vi "[FPGA] DeltaSig and SARs Main.vi"() -> ()   [LabVIEW 2025]
doc: "This VI provides a template for customizing a waveform acquisition using delta-sigma based NI C Series analog input smodules."
uses:
  <vilib>/eio/EIONode/EIONode.xnode
  <vilib>/eio/EIOPropertyNode/EIOPropertyNode.xnode
  <vilib>/rvi/DataTransferAndStorage/Container/XNode/niFpgaContainer.xnode
  <vilib>/rvi/eio/common/nirviEmuTemplateMethod_errors.vi
  <vilib>/LabVIEW Targets/FPGA/cRIO/shared/nicrio_DsaDataRateApi/_nicrio_9234GetDataRate131.vi
  <vilib>/rvi/interface/RandomDataEmulation/nirviRandomDataFpgaReadWriteTemplate.vi
  <vilib>/LabVIEW Targets/FPGA/cRIO/shared/nicrio_ModuleControls/nicrio_cRIO-9234_DataRatesRing2.ctl
  <vilib>/rvi/eio/common/nirviEmuTemplatePropertyGet_errors.vi
  <vilib>/rvi/eio/common/nirviEmuTemplatePropertyGet_noerrors.vi
  <vilib>/rvi/eio/common/nirviEmuTemplatePropertySet_errors.vi
  <vilib>/rvi/eio/common/nirviEmuTemplatePropertySet_noerrors.vi
panel:
  out "oclk freq":u32
  out "oclk div":u32
  out "oclk mult":u32
  in  "data rate (S/s)":u32
  in  "Chan Scale Array":sgl[](array[numeric])=[0.0, 0.0, 0.0, 0.0, 0.0, 0.0, 0.0, 0.0, 0.0, 0.0, 0.0, 0.0, 0.0, 0.0, 0.0, 0.0, 0.0, 0.0, 0.0, 0.0, 0.0, 0.0, 0.0, 0.0, 0.0, 0.0, 0.0, 0.0, 0.0, 0.0, 0.0, 0.0, 0.0, 0.0, 0.0, 0.0, 0.0, 0.0, 0.0, 0.0]
  out "Chan Count":bool
  out "Acq Loop Ticks":u32
  out "FPGA Error":errorcluster
  out "Module Underflow":bool
  out "Finished":bool
  in  "Number of Channels":i32=4
  in  "Samps per Chan [Finite]":i32=5120
  out "First Read":bool
  in  "Acquisition Type":enum16{"Finite Samples", "Continuous Samples"}(ring)
  out "DMA FIFO Full":bool
  in  "stop":bool
  # "Array size fixed at 40\nelements but may be \nexpanded if needed"
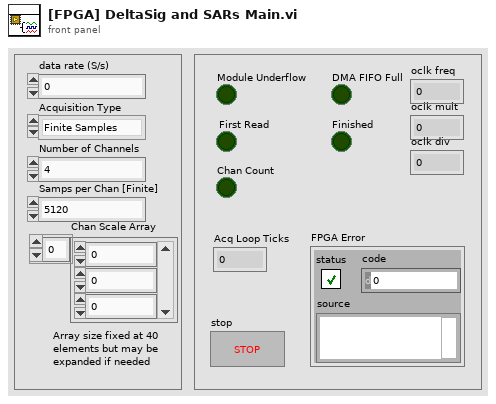
[diagram p1: front panel]
types:
  T1 = typedef "nicrio_cRIO-9234_DataRatesRing2.ctl" = u8
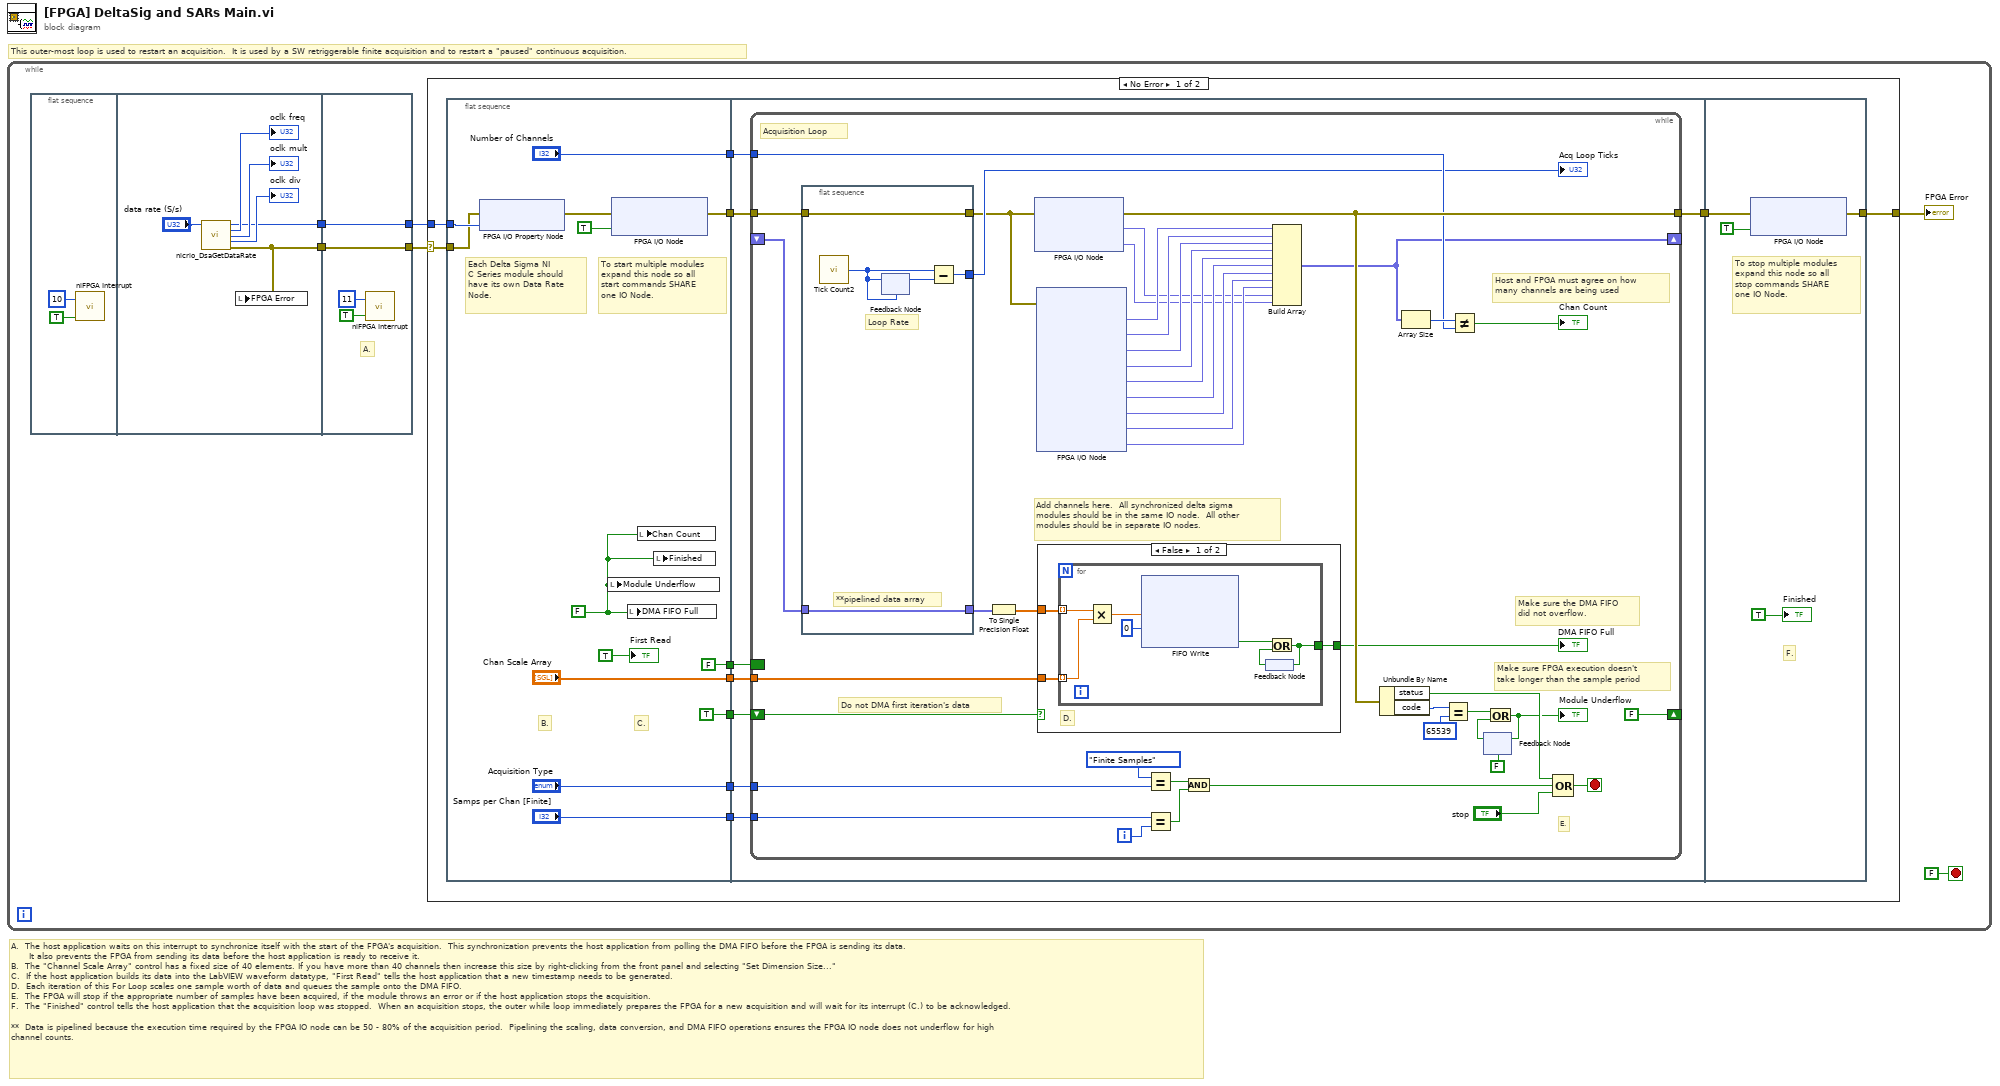
[diagram p0: block diagram]
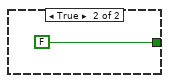
[diagram p2: hidden frame]
diagram:
  # "A.  The host application waits on this interrupt to synchronize itself with the start of the FPGA's acquisition.  This synchronization prevents the host application from polling the DMA FIFO before the FPGA is sending its data.\n      It also prevents the FPGA from sending its data before the host application is ready to receive it.\nB.  The \"Channel Scale Array\" control has a fixed size of 40 elements. If you have more than 40 channels then increase this size by right-clicking from the front panel and selecting \"Set Dimension Size...\"\nC.  If the host application builds its data into the LabVIEW waveform datatype, \"First Read\" tells the host application that a new timestamp needs to be generated.\nD.  Each iteration of this For Loop scales one sample worth of data and queues the sample onto the DMA FIFO.  \nE.  The FPGA will stop if the appropriate number of samples have been acquired, if the module throws an error or if the host application stops the acquisition.  \nF.  The \"Finished\" control tells the host application that the acquisition loop was stopped.  When an acquisition stops, the outer while loop immediately prepares the FPGA for a new acquisition and will wait for its interrupt (C.) to be acknowledged.\n\n**  Data is pipelined because the execution time required by the FPGA IO node can be 50 - 80% of the acquisition period.  Pipelining the scaling, data conversion, and DMA FIFO operations ensures the FPGA IO node does not underflow for high\nchannel counts."
  # "This outer-most loop is used to restart an acquisition.  It is used by a SW retriggerable finite acquisition and to restart a \"paused\" continuous acquisition."
  n1 = while {
    stop <- FALSE stop-if-true
    n2 = flat-sequence {
      tunnel: [w10] -> w2
      tunnel: [w11] -> w1
      tunnel: [w18] -> w3
      tunnel: [w15] -> w4
      tunnel: w2 -> [w15]
      tunnel: w1 -> [w18]
      frame #0 {
        n3 = call <vilib>:"niFPGA Interrupt.vi"("Wait Until Cleared (F)"=TRUE ("Wait Until Cleared"), "IRQ Number (0)"=u8 10 ("IRQ Number")) -> ()  [unwired: 1 in]
      }
      frame #1 {
        n4 = call-poly <vilib>:"nicrio_DsaGetDataRate.vi"("data rate (S/s)"="data rate (S/s)") -> ("data rate"=w11:T1, "oclk freq"=→"oclk freq":u32, "oclk mult"=→"oclk mult":u32, "oclk div"=→"oclk div":u32, "error out"=w10:errorcluster)  [unwired: 10 in]
        n5 = local write "FPGA Error"(w10) -> ()
      }
      frame #2 {
        # "A."
        n6 = call <vilib>:"niFPGA Interrupt.vi"("Wait Until Cleared (F)"=TRUE ("Wait Until Cleared"), "IRQ Number (0)"=u8 11 ("IRQ Number")) -> ()  [unwired: 1 in]
      }
    }
    n7 = case shown="No Error" w4 {
      selector: w4 -> [w19 w113]
      tunnel: [w21 w113] -> w5
      tunnel: w3 -> [w20 _]
      frame No Error {
        n8 = flat-sequence {
          tunnel: [w42] -> w29
          tunnel: ["Chan Scale Array"] -> w28
          tunnel: ["Acquisition Type"] -> w27
          tunnel: ["Samps per Chan [Finite]"] -> w26
          tunnel: ["Number of Channels"] -> w25
          tunnel: [TRUE ("t")] -> w24
          tunnel: [FALSE] -> w23
          tunnel: w20 -> [w31]
          tunnel: w19 -> [w30]
          tunnel: w29 -> [w49]
          tunnel: w28 -> [w48]
          tunnel: w27 -> [w46]
          tunnel: w26 -> [w45]
          tunnel: w25 -> [w50]
          tunnel: w24 -> [w47]
          tunnel: [w44] -> w22
          tunnel: w23 -> [w43]
          tunnel: w22 -> [w110]
          tunnel: [w109] -> w21
          frame #0 {
            w39 = FALSE ("Module Underflow")
            # "To start multiple modules\nexpand this node so all\nstart commands SHARE\none IO Node."
            # "C."
            # "B."
            # "Each Delta Sigma NI \nC Series module should \nhave its own Data Rate \nNode."
            n9 = xnode "FPGA I/O Property Node"("error in"=w30, "Data Rate"=w31) -> ("error out"=w38:errorcluster)  [unwired: 1 in, 1 out]
            n10 = local write "Module Underflow"(w39) -> ()
            n11 = xnode "FPGA I/O Node"("error in"=w38, "Mod7/Start"=TRUE ("Mod1/Start")) -> ("error out"=w42:errorcluster)  [unwired: 1 in, 1 out]
            n12 = local write "DMA FIFO Full"(w39) -> ()
            n13 = local write "Chan Count"(w39) -> ()
            n14 = local write "Finished"(w39) -> ()
            "First Read" <- TRUE ("First Read")
          }
          frame #1 {
            n15 = while {
              tunnel: w49 -> [w80]
              tunnel: [w85] -> w44
              tunnel: w46 -> [w87]
              tunnel: w45 -> [w86]
              shift-right: [w65] -> _
              shift-left: _ -> [w77]
              tunnel: w50 -> [w82]
              tunnel: w48 -> [w78]
              shift-right: [FALSE ("t")] -> _
              shift-left: w47 -> [w76]
              border: w43 -> [_]
              i -> [w74]
              stop <- w90 stop-if-true
              # "Add channels here.  All synchronized delta sigma\nmodules should be in the same IO node.  All other\nmodules should be in separate IO nodes."
              # "Do not DMA first iteration's data"
              # "Acquisition Loop"
              # "E."
              # "Host and FPGA must agree on how \nmany channels are being used"
              # "Make sure the DMA FIFO\ndid not overflow."
              # "Make sure FPGA execution doesn't\ntake longer than the sample period"
              n16 = flat-sequence {
                tunnel: [w108] -> w62
                tunnel: w80 -> [w108]
                tunnel: [w105] -> w79
                tunnel: w77 -> [w104]
                tunnel: [w104] -> w64
                frame #0 {
                  # "**pipelined data array"
                  # "Loop Rate"
                  n17 = call "Tick Count2"() -> ("Tick Count(Ticks)"=w107:u32)
                  n18 = feedback-in #1(w107) -> ()
                  n19 = feedback #1(w107) -> (w106:u32)
                  n20 = Subtract(x=w107, y=w106) -> (x-y=w105:u32)
                }
              }
              n21 = To Single Precision Float(number=w64) -> (single precision float=w63:sgl[])
              n22 = xnode "FPGA I/O Node"("error in"=w62) -> ("error out"=w85:errorcluster, "Mod7/AI0"=w52:fxp<+/-,24,4>, "Mod7/AI1"=w51:fxp<+/-,24,4>)  [unwired: 2 in, 2 out]
              n23 = xnode "FPGA I/O Node"("error in"=w62) -> ("Mod4/AI0"=w61:fxp<+/-,26,5>, "Mod4/AI1"=w60:fxp<+/-,26,5>, "Mod4/AI2"=w59:fxp<+/-,26,5>, "Mod4/AI3"=w58:fxp<+/-,26,5>, "Mod5/AI0"=w57:fxp<+/-,20,5>, "Mod5/AI1"=w56:fxp<+/-,20,5>, "Mod5/AI2"=w55:fxp<+/-,20,5>, "Mod5/AI3"=w54:fxp<+/-,20,5>, "Mod6/AI0"=w53:fxp<+/-,16,7>)  [unwired: 9 in, 10 out]
              n24 = case shown="False" w76 {
                tunnel: [w95 FALSE] -> w84
                tunnel: w78 -> [w94 _]
                tunnel: w63 -> [w93 _]
                frame False {
                  # "D."
                  n25 = for {
                    tunnel: [w100] -> w95
                    tunnel: w93 -> [w98] mode=indexing
                    tunnel: w94 -> [w97] mode=indexing
                    n26 = Multiply(x=w98, y=w97) -> (x*y=w96:sgl)
                    n27 = xnode ("FIFO Write")("Element"=w96, "Timeout"=0) -> ("Timed Out?"=w102:bool)  [unwired: 1 in, 1 out]
                    n28 = feedback #2() -> (w101:bool)
                    n29 = Or(x=w102, y=w101) -> (x .or. y?=w100:bool)
                    n30 = feedback-in #2(w100) -> ()
                  }
                }
                frame True {
                }
              }
              "DMA FIFO Full" <- w84
              n31 = Equal?(x=enum16{"Finite Samples", "Continuous Samples"}."Finite Samples" ("y"), y=w87) -> (x = y?=w68:bool)
              n32 = Equal?(x=w86, y=w74) -> (x = y?=w67:bool)
              n33 = And(x=w68, y=w67) -> (x .and. y?=w66:bool)
              n34 = Build Array(w61, w60, w59, w58, w57, w56, w55, w54, w53, w52, w51) -> (w65:fxp<+/-,28,7>[])
              n35 = Unbundle By Name(w85) -> ("status"=w73:bool, "code"=w88:i32)
              n36 = Array Size(array=w65) -> (size(s)=w83:i32)
              n37 = Equal?(x=w88, y=65539) -> (x = y?=w70:bool)
              n38 = Not Equal?(x=w83, y=w82) -> (x != y?=→"Chan Count":bool)
              n39 = feedback #3(FALSE) -> (w72:bool)
              n40 = Or(x=w70, y=w72) -> (x .or. y?=w69:bool)
              "Module Underflow" <- w69
              n41 = feedback-in #3(w69) -> ()
              n42 = Compound Arithmetic op=OR(w73, w66, "stop") -> (w90:bool)
              "Acq Loop Ticks" <- w79
            }
          }
          frame #2 {
            # "To stop multiple modules\nexpand this node so all\nstop commands SHARE\none IO Node."
            # "F."
            n43 = xnode "FPGA I/O Node"("error in"=w110, "Mod7/Stop"=TRUE ("Mod1/Stop")) -> ("error out"=w109:errorcluster)  [unwired: 1 in, 1 out]
            "Finished" <- TRUE ("Finished")
          }
        }
      }
      frame Error {
      }
    }
    "FPGA Error" <- w5
  }
